vi "makeDecisions.vi"(8 "error in (no error)":errorcluster, 10 "model":refnum<class "Model.lvclass">, 11 "EndingCycleState in":refnum<class "EndingCycleState.lvclass">) -> (0 "error out":errorcluster, 2 "model 2":refnum<class "Model.lvclass">, 3 "EndingCycleState out":refnum<class "EndingCycleState.lvclass">)   [LabVIEW 2013, in "EndingCycleState.lvclass"]
uses:
  EndingCycleState.lvclass
  Model/Model/Model.lvclass
  TestingState/TestingState.lvclass
  Typedefs/StateSelector.ctl
  Typedefs/AITDTTypedefs.lvlib
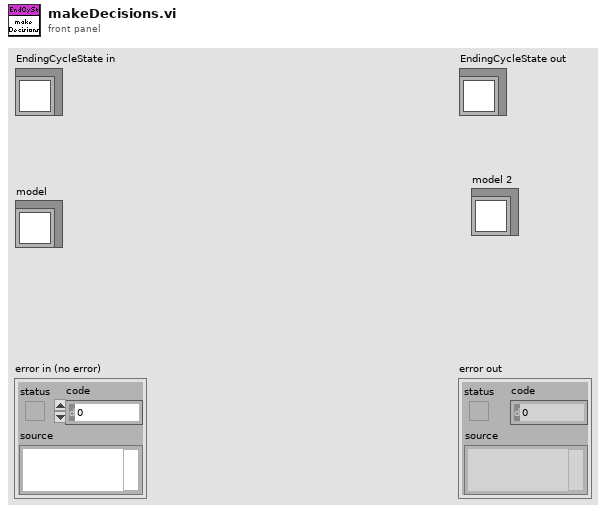
[diagram p1: front panel]
types:
  T1 = typedef "AITDTTypedefs.lvlib/StateSelector.ctl" = enum16{"AwaitingSetpointAcknowledgmentState", "EndingCycleState", "FaultState", "OffState", "PausingState", "RequestingNewSetpointState", "SamplingState", "SettlingState", "SoakingState", "StabilizingState", "StandbyState", "StoppedState", "TransitioningTemperatureState"}
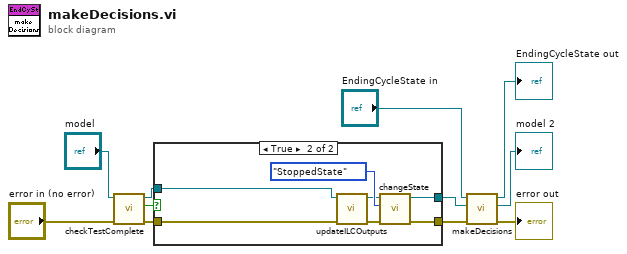
[diagram p0: block diagram]
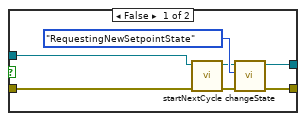
[diagram p2: hidden frame]
diagram:
  n1 = call "checkTestComplete.vi"("error in (no error)"="error in (no error)", "Model in"="model") -> ("error out"=w4:errorcluster, "testCompleteIsTrue"=w1:bool, "Model out"=w6:refnum<class "Model.lvclass">)  [unwired: 7 in]
  n2 = case shown="True" w1 {
    tunnel: w6 -> [w18 w20]
    tunnel: w4 -> [w16 w19]
    tunnel: [w15 w24] -> w3
    tunnel: [w17 w23] -> w2
    frame False {
      n3 = call "startNextCycle.vi"("error in (no error)"=w16, "Model in"=w18) -> ("error out"=w12:errorcluster, "Model out"=w13:refnum<class "Model.lvclass">)  [unwired: 8 in]
      n4 = call "changeState.vi"("error in (no error)"=w12, "State:"=StateSelector."RequestingNewSetpointState", "Model in"=w13) -> ("error out"=w15:errorcluster, "Model out"=w17:refnum<class "Model.lvclass">)  [unwired: 7 in]
    }
    frame True {
      n5 = call "updateILCOutputs.vi"("error in (no error)"=w19, "Model in"=w20) -> ("error out"=w21:errorcluster, "Model out"=w22:refnum<class "Model.lvclass">)  [unwired: 8 in]
      n6 = call "changeState.vi"("error in (no error)"=w21, "State:"=StateSelector."StoppedState", "Model in"=w22) -> ("error out"=w24:errorcluster, "Model out"=w23:refnum<class "Model.lvclass">)  [unwired: 7 in]
    }
  }
  n7 = call-parent "makeDecisions.vi"("error in (no error)"=w3, "model"=w2, "EnabledState in"="EndingCycleState in") -> ("error out"=→"error out":errorcluster, "model 2"=→"model 2":refnum<class "Model.lvclass">, "EnabledState out"=→"EndingCycleState out":refnum<class "EndingCycleState.lvclass">)  [unwired: 6 in]
